vi "RobotConstants.vi"() -> (0 "Arena Width (m)":dbl, 1 "Arena Height (m)":dbl, 2 "Robot Width (m)":dbl=0.71, 3 "atan((width/2) / (length/2))":dbl=0.5662076900747014, 4 "Robot Length (m)":dbl=1.117)   [LabVIEW 2015, in "Localization Mockup.lvlib"]
uses:
  Localization Mockup.lvlib
panel:
  in  "Arena Height (m)":dbl=3.78
  in  "Arena Width (m)":dbl=7.38
  in  "Robot Length (m)":dbl=1.117
  in  "Robot Width (m)":dbl=0.71
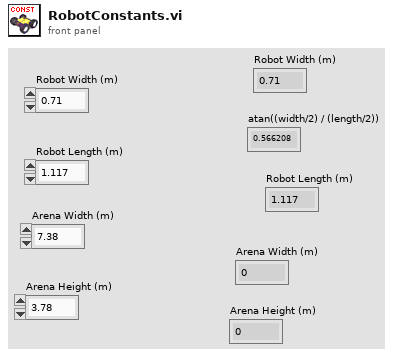
[diagram p1: front panel]
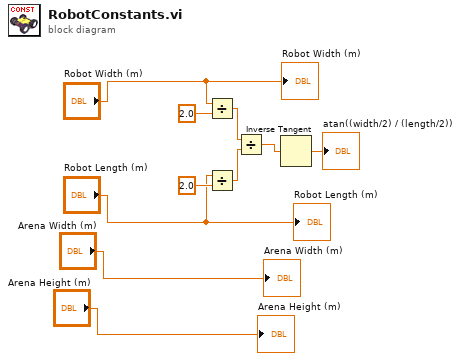
[diagram p0: block diagram]
diagram:
  n1 = Divide(x="Robot Width (m)", y=2.0) -> (x/y=w7:dbl)
  n2 = Divide(x="Robot Length (m)", y=2.0) -> (x/y=w3:dbl)
  n3 = Divide(x=w7, y=w3) -> (x/y=w6:dbl)
  n4 = Inverse Tangent(1:w6) -> (0:→"atan((width/2) / (length/2))":dbl)
  "Robot Width (m)" <- "Robot Width (m)"
  "Robot Length (m)" <- "Robot Length (m)"
  "Arena Width (m)" <- "Arena Width (m)"
  "Arena Height (m)" <- "Arena Height (m)"
